vi "Dashboard Main.vi"() -> ()   [LabVIEW 2017]
uses:
  <vilib>/Utility/miscctls.llb/LVRowAndColumnTypeDef.ctl
  <vilib>/event_ctls.llb/eventvkey.ctl
  <vilib>/Rock Robotics/Network Tables/NT Read Numeric Array.vi
  <vilib>/Rock Robotics/Network Tables/NT Read Boolean.vi
  <vilib>/Rock Robotics/WPI/Dashboard/WPI_DashboardLogging Global.vi
  <vilib>/vision/NI_Vision_Development_Module.lvlib
panel:
  in  "Camera Settings Right":T1={"Frame Rate"=30, "Compression"=30, "Size"=1, "DB Camera Config"=FALSE} {"Frame Rate" scale=1.0..30.0; "Compression" scale=100.0..-1.0; "Size" items=["640x480", "320x240", "160x120"]}
  in  "Camera Name Right":string(combo)="No Camera Selection"
  out "Camera Info":cluster{"Mbps LED":bool, "Mbps":dbl, "fps":dbl} {"fps" format="%#.1g"; "Mbps" format="%#.1g"}
  in  "Camera Settings":T1={"Frame Rate"=30, "Compression"=30, "Size"=1, "DB Camera Config"=FALSE} {"Frame Rate" scale=1.0..30.0; "Compression" scale=100.0..-1.0; "Size" items=["640x480", "320x240", "160x120"]}
  in  "TCP":refnum<k5>
  in  "Rec Mode":enum32{"Stop", "Record", "Playback"}(radio)
  out "Robot IP":string
  out "Image Message":string="Timeout in Camera Communications"
  in  "Dashboard Tab":T2(tab)
  in  "Select Auto":string(combo)="Select Autonomous ..."
  out "NT Connection":bool
  out "MotorChart R":cluster{"Numeric":dbl, "Numeric":dbl}(graph)
  out "MotorChart L":cluster{"Numeric":dbl, "Numeric":dbl}(graph)
  out "MotorSliders R":cluster{"MotorSlide1":dbl, "MotorSlide2":dbl} {"MotorSlide2" scale=-1.0..1.0 scale format="%#_2e"; "MotorSlide1" scale=-1.0..1.0 scale format="%#_2e"}
  out "MotorSliders L":cluster{"MotorSlide1":dbl, "MotorSlide2":dbl} {"MotorSlide2" scale=-1.0..1.0 scale format="%#_2e"; "MotorSlide1" scale=-1.0..1.0 scale format="%#_2e"}
  out "Gyro":dbl(knob) scale=0.0..360.0
  out "JS1 Z":dbl(slide) scale=-1.0..1.0 scale format="%#_2e"
  out "JS1 Graph":cluster{"X":dbl, "Y":dbl}[](graph)
  out "JS1 Buttons":T3
  out "JS2 Z":dbl(slide) scale=-1.0..1.0 scale format="%#_2e"
  out "JS2 Graph":cluster{"X":dbl, "Y":dbl}[](graph)
  out "JS2 Buttons":T3
  out "Mode":T4(ring)=enum."Auto Disabled"
  out "Camera Image Right":T5(plugin-control)
  in  "DB/String 9":string
  in  "DB/String 8":string
  in  "DB/String 7":string
  in  "DB/String 6":string
  in  "DB/String 5":string
  in  "DB/String 4":string
  in  "DB/String 3":string
  in  "DB/String 2":string
  in  "DB/String 1":string
  in  "DB/String 0":string
  in  "DB/Slider 0":dbl(slide) scale=0.0..5.0
  in  "DB/Slider 1":dbl(slide) scale=0.0..5.0
  in  "DB/Slider 2":dbl(slide) scale=0.0..5.0
  in  "DB/Slider 3":dbl(slide) scale=0.0..5.0
  out "DB/LED 3":bool
  out "DB/LED 2":bool
  out "DB/LED 1":bool
  out "DB/LED 0":bool
  in  "DB/Button 3":bool
  in  "DB/Button 2":bool
  in  "DB/Button 1":bool
  in  "DB/Button 0":bool caption="New Name"
  out "UseLeftEncoder":bool
  out "RDrive Encoder":dbl
  out "Flip Active":bool
  in  "BackCamera Rotate":sgl min=-360 max=360 step=1 format="%#_3g"
  in  "FrontCamera Rotate":sgl min=-360 max=360 step=1 format="%#_3g"
  out "Arm Sensor":bool
  out "Belly Sensor":bool
  out "Arm Encoder":dbl
  out "Arm Switch":bool
  out "LDrive Encoder":dbl
  in  "Test Slider":dbl(slide) scale=0.0..100.0 scale format="%#_3g"
  in  "On/Off":bool caption="Solenoid"
  in  "Test Name":u16(ring) items=["Select the test to run..."]
  in  "Test Tree":string(tree)
  in  "Motor":cluster{"Value":dbl, "Enable":bool} {"Value" scale=-1.0..1.0 scale format="%#_3g"}
  out "Progress":T6 {"Test Progress" scale=0.0..100.0}
  in  "Rev/Fwd":cluster{"Forward":bool, "Reverse":bool}
  in  "Test Ring":u16(ring) items=["Monochrome", "Color"]
  out "Cmd Status":string
  in  "Execute Command":bool
  in  "Command Params":string[][](table)
  in  "Command Selection":i32(listbox)
  in  "CheckList":i32(listbox)
  out "Tree":string(tree)
  out "Camera Image":T5(plugin-control)
  out "Background":bool
  in  "Camera Name":string(combo)="No Camera Selection"
  # "HW"
  # "HW"
  # "Joysticks"
  # "Drive Motors"
  # "Front"
  # "Right"
  # "Left"
  # "Back"
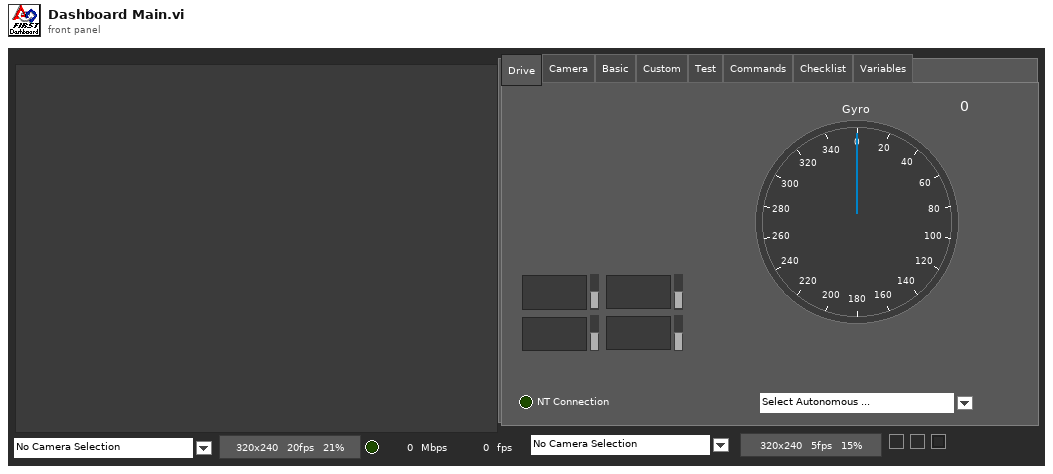
[diagram p1: front panel]
types:
  T1 = cluster{"Frame Rate":i32, "Compression":i32, "Size":u16, "DB Camera Config":bool}
  T2 = enum32{"Drive", "Camera", "Basic", "Custom", "Test", "Commands", "Checklist", "Variables"}
  T3 = cluster{bool, bool, bool, bool, bool, bool, bool, bool, bool, bool, bool, bool}
  T4 = enum8{"Tele-Op Disabled", "Tele-Op Enabled", "Auto Disabled", "Auto Enabled", "Test Disabled", "Test Enabled", "Disconnected", "No Code", "E-Stop"}
  T5 = typedef "IMAQ Image.ctl" = refnum<image>
  T6 = cluster{"Test Progress":u8, "Test Progress Text":string}
  T7 = cluster{"Save Path":path, "Interval (s)":dbl, "Keep":i32}
  T8 = typedef "Image Type" = u32
  T9 = cluster{"IDs":cluster{"RPC field ID":u16, "Unique ID":u16}, "String":string}
  T10 = cluster{string, string, "Saved DB Images Info":cluster{"Save Path":path, "Interval (s)":dbl, "Keep":i32}}
  T11 = cluster{"Camera Image":refnum<vi>, "Dashboard Tab":refnum<vi>, "Background":refnum<vi>, "Rec Mode":refnum<vi>, "Test Slider":refnum<vi>, "On/Off ":refnum<vi>, "Test Ring":refnum<vi>, "Rev/Fwd":refnum<vi>, "Test Name":refnum<vi>, "Motor":refnum<vi>, "Progress":refnum<vi>, "CheckList":refnum<vi>, "Tree":refnum<vi>, "Test Tree":refnum<vi>, "Command Params":refnum<vi>, "Command Selection":refnum<vi>, "Execute Command":refnum<vi>, "Cmd Status":refnum<vi>, "Camera Settings":refnum<vi>, "Camera Name":refnum<vi>, "Camera Info":refnum<vi>, "Camera Settings Right":refnum<vi>, "Camera Name Right":refnum<vi>, "Camera Image Right":refnum<vi>}
  T12 = cluster{"Error Strings":string, "Disable Counts":cluster{u16, u16}, "Rail Faults":cluster{u16, u16, u16}, "Robot IP":string, "DB Mode":u8, "Event Info":cluster{"Name":string, "Type":u8, "Number":u16, "Replay":u8}}
  T13 = cluster{"Storage":cluster{"Disk Free":u64, "RAM Block":u32, "RAM free":u32}, "CPU Utilization":cluster{"CPU % ISR":sgl, "CPU % Time Crit":sgl, "CPU % Timed Str":sgl, "CPU % High":sgl, "CPU % Above":sgl, "CPU % Normal":sgl, "CPU % Low":sgl}, "CAN":cluster{"% Bus Utilization":sgl, "Bus Off Cnt":u32, "TX_FIFO Full Cnt":u32, "Receive Error Cnt":u8, "Transmit Error Cnt":u8}, "HID":cluster{"HID Outputs":u32, "Rumble Low":u16, "Rumble High":u16}[]}
  T14 = cluster{"Status bits":cluster{"Test Mode":bool, "Autonomous":bool, "Enabled":bool, "Code Start":bool, "Brownout":bool, "Reserved 2":bool, "Reserved 3":bool, "E-Stop":bool}, "Code Trace":cluster{"Disabled":bool, "TeleOp":bool, "Auto":bool, "Test":bool}, "Controller Type":enum16{"unknown", "cRIO", "roboRio"}, "Code?":enum16{"unknown", "noCode", "code"}, "Battery V":dbl}
  T15 = cluster{"Control Bits":cluster{"TestMode":bool, "Autonomous":bool, "Enabled":bool, "FMS Present":bool, bool, bool, bool, "E-Stop":bool}, "Team Station ":u8, "Countdown":sgl, "Joystick Values":cluster{"Axes":dbl[], "Buttons":bool[], "POVs":i16[]}[]}
  T16 = cluster{"Axes":dbl[], "Buttons":bool[], "POVs":i16[]}[]
  T17 = cluster{"Axes":dbl[], "Buttons":bool[], "POVs":i16[]}
  T18 = cluster{"Buttons[0]":bool, "Buttons[1]":bool, "Buttons[2]":bool, "Buttons[3]":bool, "Buttons[4]":bool, "Buttons[5]":bool, "Buttons[6]":bool, "Buttons[7]":bool, "Buttons[8]":bool, "Buttons[9]":bool, "Buttons[10]":bool, "Buttons[11]":bool}
  T19 = cluster{"Camera Name Right":string, string, "Saved DB Images Info":cluster{"Save Path":path, "Interval (s)":dbl, "Keep":i32}}
  T20 = cluster{"Operation":enum16{"Update", "Clear"}, "Color Box":u32}[]
  T21 = typedef "eventvkey.ctl" = enum16{"ASCII", "Enter", "Return", "Shift", "Ctrl", "Alt", "Cmd", "Opt", "Caps", "NumLock", "Clear", "Break", "Up", "Down", "Left", "Right", "Insert", "Delete", "Home", "End", "PageUp", "PageDown", "Escape", "Help", "Pause", "ScrollLock", "F1", "F2", "F3", "F4", "F5", "F6", "F7", "F8", "F9", "F10", "F11", "F12", "F13", "F14", "F15", "F16", "F17", "F18", "F19", "F20", "F21", "F22", "F23", "F24", "Play", "VolumeUp", "VolumeDown", "Mute", "Two Byte Char"}
  T22 = cluster{"Image Size":bool, "Image Type":bool, "Pixel Value":bool, "ROI Information":bool, "Zoom Factor":bool}
  T23 = cluster{"Operation":enum16{"Update", "Clear"}, "Color Box":u32}
  T24 = typedef "LVRowAndColumnTypeDef.ctl" = cluster{"Row":i32, "Column":i32}
  T25 = cluster{"Shift":bool, "Ctrl":bool, "Alt":bool, "Cmd":bool, "Opt":bool}
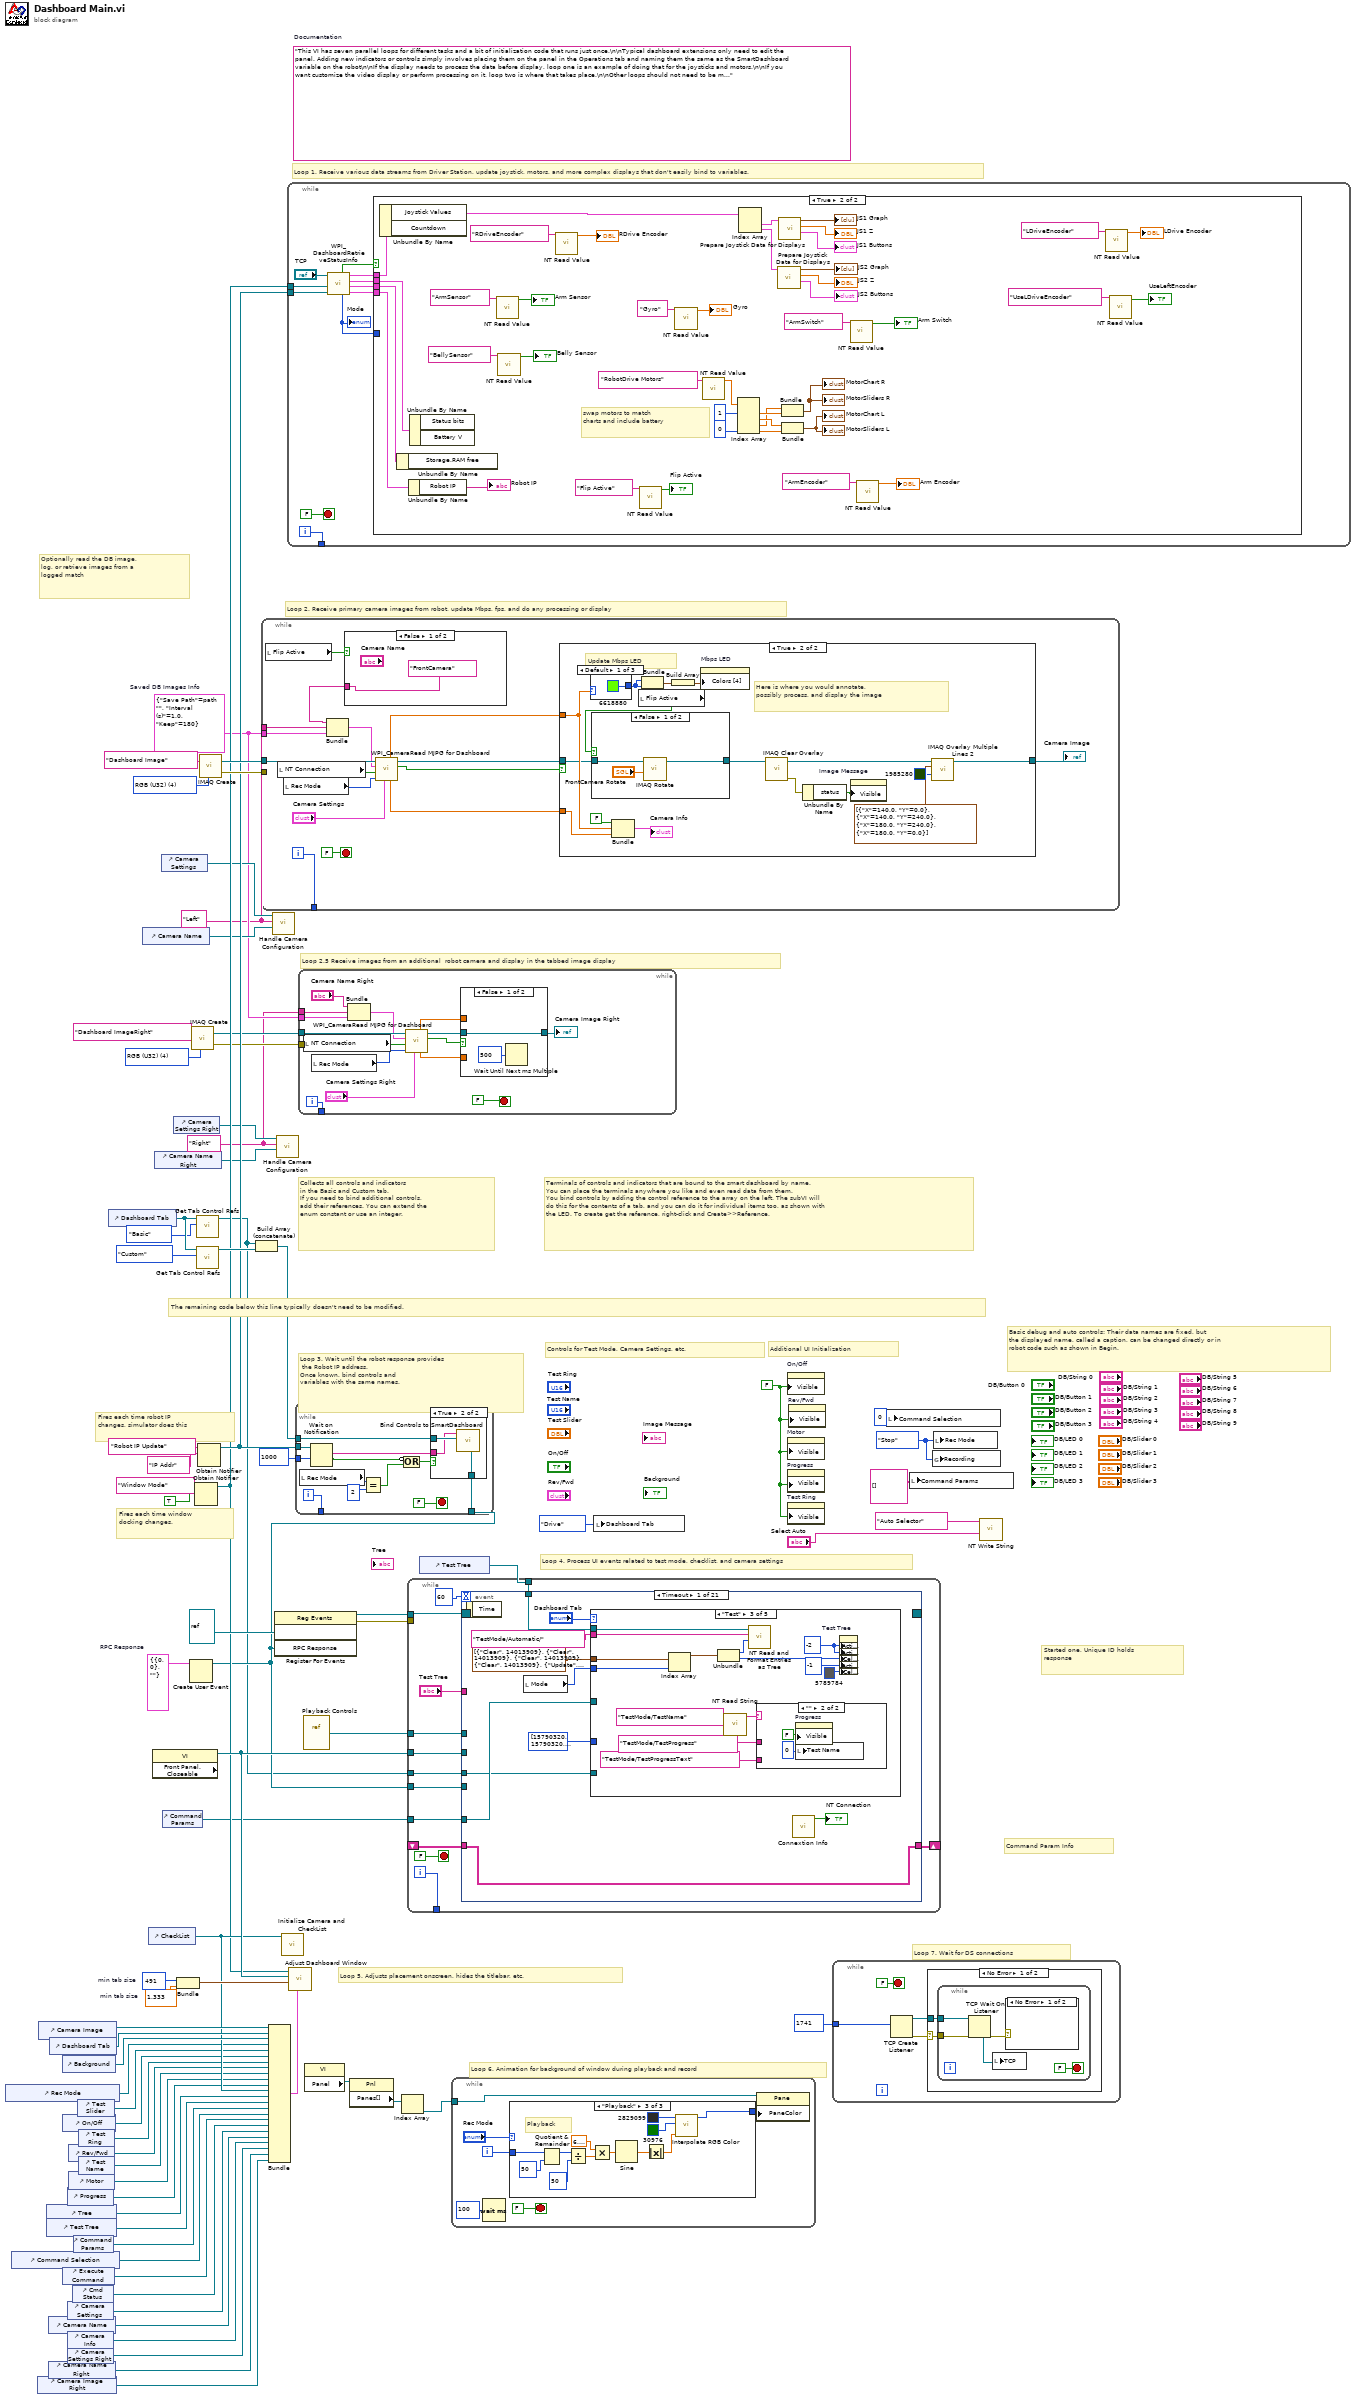
[diagram p0: block diagram]
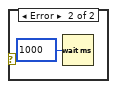
[diagram p3: hidden frame]
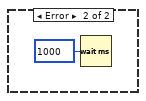
[diagram p4: hidden frame]
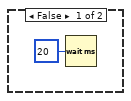
[diagram p5: hidden frame]
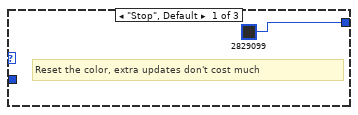
[diagram p6: hidden frame]
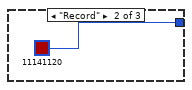
[diagram p7: hidden frame]
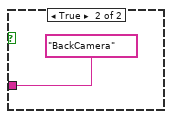
[diagram p9: hidden frame]
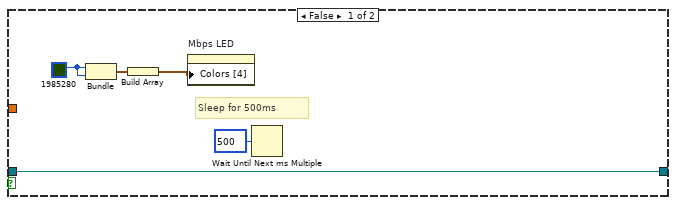
[diagram p10: hidden frame]
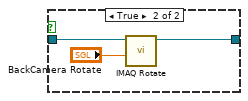
[diagram p11: hidden frame]
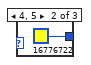
[diagram p12: hidden frame]
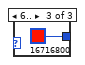
[diagram p13: hidden frame]
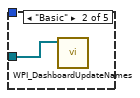
[diagram p15: hidden frame]
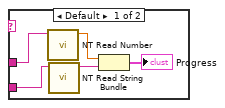
[diagram p16: hidden frame]
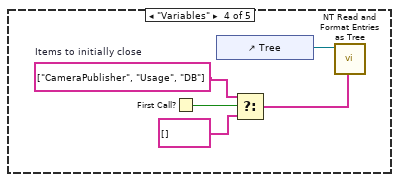
[diagram p17: hidden frame]
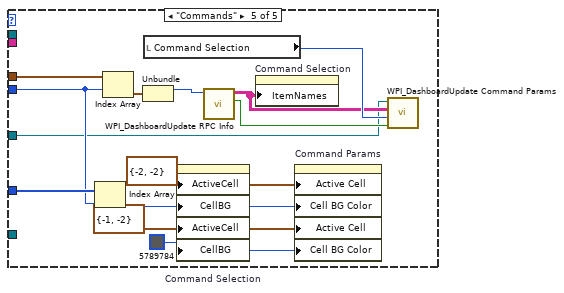
[diagram p18: hidden frame]
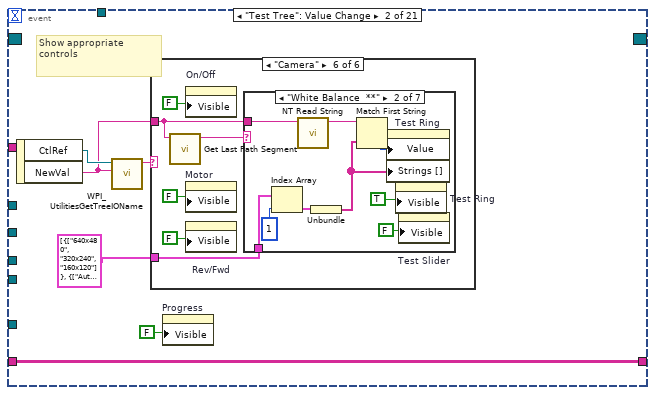
[diagram p19: hidden frame]
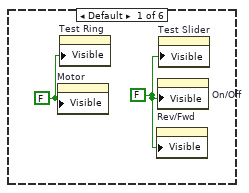
[diagram p20: hidden frame]
diagram:
  w4 = T7 {"Save Path"=path "", "Interval (s)"=1.0, "Keep"=180}  # Saved DB Images Info
  w3 = "Right"
  w2 = "Left"
  w14 = T8 4 items=["Grayscale (U8)", "Grayscale (I16)", "Grayscale (SGL)", "Complex (CSG)", "RGB (U32)", "HSL (U32)", "RGB (U64)"] ("Image Type")
  w29 = T9 {"IDs"={"RPC field ID"=0, "Unique ID"=0}, "String"=""}  # RPC Response
  w52 = 491  # min tab size
  w51 = 1.333  # min tab size
  w59 = enum32{"Stop", "Record", "Playback"}."Stop" ("Rec Mode")
  w36 = FALSE ("Visible")
  (unwired) "This VI has seven parallel loops for different tasks and a bit of initialization code that runs just once.\n\nTypical dashboard extensions only need to edit the panel. Adding new indicators or controls simply involves placing them on the panel in the Operations tab and naming them the same as the SmartDashboard variable on the robot\n\nIf the display needs to process the data before display, loop one is an example of doing that for the joysticks and motors.\n\nIf you want customize the video display or perform processing on it, loop two is where that takes place.\n\nOther loops should not need to be modified. They are pretty standard, and document the task they perform."  # Documentation
  w76 = T8 4 items=["Grayscale (U8)", "Grayscale (I16)", "Grayscale (SGL)", "Complex (CSG)", "RGB (U32)", "HSL (U32)", "RGB (U64)"] ("Image Type")
  # "Optionally read the DB image,\nlog, or retrieve images from a\nlogged match"
  # "Loop 2.5 Receive images from an additional  robot camera and display in the tabbed image display"
  # "Command Param Info"
  # "Started one, Unique ID holds\nresponse"
  # "Loop 7. Wait for DS connections"
  # "Basic debug and auto controls: Their data names are fixed, but\nthe displayed name, called a caption, can be changed directly or in\nrobot code such as shown in Begin."
  # "Controls for Test Mode, Camera Settings, etc."
  # "Additional UI Initialization"
  # "Loop 6. Animation for background of window during playback and record"
  # "Fires each time robot IP\nchanges, simulator does this"
  # "Fires each time window\ndocking changes."
  # "Collects all controls and indicators\nin the Basic and Custom tab.\nIf you need to bind additional controls,\nadd their references. You can extend the\nenum constant or use an integer."
  # "The remaining code below this line typically doesn't need to be modified."
  # "Loop 4. Process UI events related to test mode, checklist, and camera settings"
  # "Terminals of controls and indicators that are bound to the smart dashboard by name.\nYou can place the terminals anywhere you like and even read data from them.\nYou bind controls by adding the control reference to the array on the left. The subVI will\ndo this for the contents of a tab, and you can do it for individual items too, as shown with\nthe LED. To create get the reference, right-click and Create>>Reference."
  # "Loop 3. Wait until the robot response provides\n the Robot IP address.\nOnce known, bind controls and\nvariables with the same names."
  # "Loop 5. Adjusts placement onscreen, hides the titlebar, etc."
  # "Loop 1. Receive various data streams from Driver Station, update joystick, motors, and more complex displays that don't easily bind to variables."
  # "Loop 2. Receive primary camera images from robot, update Mbps, fps, and do any processing or display"
  n1 = control-ref of="Rec Mode"() -> (w42:refnum<vi>)
  n2 = control-ref of="Command Selection"() -> (w28:refnum<vi>)
  n3 = control-ref of="Camera Image Right"() -> (w7:refnum<vi>)
  n4 = control-ref of="Camera Image"() -> (w54:refnum<vi>)
  n5 = control-ref of="Tree"() -> (w46:refnum<vi>)
  n6 = control-ref of="Test Tree"() -> (w45:refnum<vi>)
  n7 = control-ref of="Camera Name"() -> (w19:refnum<vi>)
  n8 = control-ref of="Camera Name Right"() -> (w8:refnum<vi>)
  n9 = control-ref of="Dashboard Tab"() -> (w53:refnum<vi>)
  n10 = control-ref of="Execute Command"() -> (w30:refnum<vi>)
  n11 = control-ref of="Background"() -> (w49:refnum<vi>)
  n12 = control-ref of="On/Off"() -> (w40:refnum<vi>)
  n13 = control-ref of="Progress"() -> (w37:refnum<vi>)
  n14 = control-ref of="Camera Settings"() -> (w20:refnum<vi>)
  n15 = control-ref of="Camera Info"() -> (w18:refnum<vi>)
  n16 = control-ref of="Camera Settings Right"() -> (w9:refnum<vi>)
  n17 = control-ref of="Rev/Fwd"() -> (w38:refnum<vi>)
  n18 = control-ref of="Motor"() -> (w43:refnum<vi>)
  n19 = control-ref of="Cmd Status"() -> (w24:refnum<vi>)
  n20 = control-ref of="Command Params"() -> (w31:refnum<vi>)
  n21 = control-ref of="Test Slider"() -> (w41:refnum<vi>)
  n22 = control-ref of="Test Ring"() -> (w39:refnum<vi>)
  n23 = control-ref of="Test Name"() -> (w44:refnum<vi>)
  n24 = control-ref of="Dashboard Tab"() -> (w57:refnum<vi>)
  n25 = control-ref of="Camera Name"() -> (w21:refnum<vi>)
  n26 = control-ref of="CheckList"() -> (w47:refnum<vi>)
  n27 = property class="VI" props=["Front Panel.Closeable"]() -> (reference out=w58:refnum<vi>)  [unwired: 2 in, 2 out]
  n28 = control-ref of="Camera Name Right"() -> (w10:refnum<vi>)
  n29 = control-ref of="Camera Settings"() -> (w22:refnum<vi>)
  n30 = control-ref of="Command Params"() -> (w23:refnum<vi>)
  n31 = control-ref of="Camera Settings Right"() -> (w11:refnum<vi>)
  n32 = Bundle("min tab size"=w52, "min tab size"=w51) -> (w50:cluster{"min tab size":i32, "min tab size":dbl})  [unwired: 1 in]
  n33 = Create User Event(user event datatype=w29) -> (user event=w25:refnum<user-event>)  [unwired: 1 in, 1 out]
  n34 = call "IMAQ Create"("Image Name"="Dashboard ImageRight", "Image Type"=w14) -> ("New Image"=w13:T5, "error out"=w12:errorcluster)  [unwired: 2 in, 1 out]
  n35 = Obtain Notifier(name (unnamed)="Window Mode", notification data type=TRUE) -> (notifier out=w34:refnum<notifier>)  [unwired: 2 in, 2 out]
  n36 = call <vilib>:"Get Tab Control Refs.vi"("Page Index"=T2."Basic" ("Dashboard Tab"), "TabControl in"=w57) -> ("ControlsOnPage"=w17:refnum<vi>[])  [unwired: 9 in]
  n37 = call <vilib>:"Get Tab Control Refs.vi"("Page Index"=T2."Custom" ("Dashboard Tab"), "TabControl in"=w57) -> ("ControlsOnPage"=w56:refnum<vi>[])  [unwired: 9 in]
  n38 = Obtain Notifier(name (unnamed)="Robot IP Update", notification data type="IP Addr" ("name (unnamed)")) -> (notifier out=w35:refnum<notifier>)  [unwired: 2 in, 2 out]
  n39 = call "IMAQ Create"("Image Name"="Dashboard Image", "Image Type"=w76) -> ("New Image"=w74:T5, "error out"=w73:errorcluster)  [unwired: 2 in, 1 out]
  n40 = Build Array (concatenate)(w17, w56) -> (w55:refnum<vi>[])
  n41 = while {
    tunnel: w74 -> [w90]
    tunnel: w73 -> [_]
    tunnel: [w91] -> _
    tunnel: w4 -> [w81]
    tunnel: w2 -> [w80]
    i -> [w91]
    stop <- FALSE stop-if-true
    n42 = local read "Flip Active"() -> (w77:bool)
    n43 = local read "NT Connection"() -> (w82:bool)
    n44 = local read "Rec Mode"() -> (w86:enum32{"Stop", "Record", "Playback"})
    n45 = case shown="False" w77 {
      tunnel: ["FrontCamera" "BackCamera"] -> w79
      frame False {
      }
      frame True {
      }
    }
    n46 = Bundle(w79, w80, "Saved DB Images Info"=w81) -> (w78:T10)  [unwired: 1 in]
    n47 = call <vilib>:"WPI_CameraRead MJPG for Dashboard.vi"("Camera Settings"="Camera Settings", "Rec Mode"=w86, "NT Connection"=w82, "Capture Info"=w78, "Refnum in"=w90) -> ("Active"=w88:bool, "Refnum out"=w89:T5, "FPS"=w87:dbl, "Bandwidth (Mbps)"=w85:dbl)  [unwired: 3 in]
    n48 = case shown="True" w88 {
      tunnel: w89 -> [w95 w102]
      tunnel: w85 -> [_ w109]
      tunnel: w87 -> [_ w110]
      tunnel: [w95 w105] -> w83
      frame False {
        w97 = u32 1985280 ("Color Box")
        # "Sleep for 500ms"
        n49 = Bundle("Color Box"=w97, "Color Box"=w97) -> (w98:cluster{"Color Box":u32, "Color Box":u32})  [unwired: 1 out]
        n50 = Build Array(w98) -> (w96:cluster{"Color Box":u32, "Color Box":u32}[])
        n51 = property on="Mbps LED" class="Bool (strict)"("Colors [4]"=w96) -> ()  [unwired: 2 in, 2 out]
        n52 = Wait Until Next ms Multiple(millisecond multiple=u32 500) -> ()  [unwired: 1 out]
      }
      frame True {
        # "Here is where you would annotate,\npossibly process, and display the image"
        # "Update Mbps LED"
        n53 = case shown="Default" w109 {
          tunnel: [u32 6618880 ("Color Box") u32 16776722 ("Color Box") u32 16716800 ("Color Box")] -> w112
          frame Default {
          }
          frame 4, 5 {
          }
          frame 6.. {
          }
        }
        n54 = Bundle(FALSE, "Bandwidth (Mbps)"=w109, "FPS"=w110) -> (→"Camera Info":cluster{bool, "Bandwidth (Mbps)":dbl, "FPS":dbl})  [unwired: 1 in]
        n55 = local read "Flip Active"() -> (w100:bool)
        n56 = case shown="False" w100 {
          tunnel: w102 -> [w118 w121]
          tunnel: [w117 w120] -> w101
          frame False {
            n57 = call "IMAQ Rotate"("Angle (degrees)"="FrontCamera Rotate", "Image Src"=w118) -> ("Image Dst Out"=w117:T5)  [unwired: 8 in, 1 out]
          }
          frame True {
            n58 = call "IMAQ Rotate"("Angle (degrees)"="BackCamera Rotate", "Image Src"=w121) -> ("Image Dst Out"=w120:T5)  [unwired: 8 in, 1 out]
          }
        }
        n59 = Bundle("Color Box"=w112, "Color Box"=w112) -> (w113:cluster{"Color Box":u32, "Color Box":u32})  [unwired: 1 out]
        n60 = Build Array(w113) -> (w111:cluster{"Color Box":u32, "Color Box":u32}[])
        n61 = property on="Mbps LED" class="Bool (strict)"("Colors [4]"=w111) -> ()  [unwired: 2 in, 2 out]
        n62 = call "IMAQ Clear Overlay"("Image"=w101) -> ("error out"=w114:errorcluster, "Image Out"=w106:T5)  [unwired: 2 in, 7 out]
        n63 = Unbundle By Name(w114) -> ("status"=w115:bool)
        n64 = property on="Image Message" class="Str"("Visible"=w115) -> ()  [unwired: 2 in, 2 out]
        n65 = call "IMAQ Overlay Multiple Lines 2"("Image"=w106, "Line End Points"=cluster{"X":dbl, "Y":dbl}[] [{"X"=140.0, "Y"=0.0}, {"X"=140.0, "Y"=240.0}, {"X"=180.0, "Y"=240.0}, {"X"=180.0, "Y"=0.0}], "Color"=u32 1985280) -> ("Image Out"=w105:T5)  [unwired: 11 in, 1 out]
      }
    }
    "Camera Image" <- w83
  }
  n66 = Bundle("Camera Image"=w54, "Dashboard Tab"=w53, "Background"=w49, "Rec Mode"=w42, "Test Slider"=w41, "On/Off"=w40, "Test Ring"=w39, "Rev/Fwd"=w38, "Test Name"=w44, "Motor"=w43, "Progress"=w37, "CheckList"=w47, "Tree"=w46, "Test Tree"=w45, "Command Params"=w31, "Command Selection"=w28, "Execute Command"=w30, "Cmd Status"=w24, "Camera Settings"=w20, "Camera Name"=w19, "Camera Info"=w18, "Camera Settings Right"=w9, "Camera Name Right"=w8, "Camera Image Right"=w7) -> (w48:T11)  [unwired: 1 in]
  n67 = call "Handle Camera Configuration.vi"("CameraNameRef"=w21, "Display Name"=w2, "ClusterRef"=w22) -> ()  [unwired: 9 in]
  n68 = register-events(refnum<vi> refnum, w25) -> (reference out=w63:refnum<event-registration>, error out=w62:errorcluster)  [unwired: 2 in]
  n69 = call "Handle Camera Configuration.vi"("CameraNameRef"=w10, "Display Name"=w3, "ClusterRef"=w11) -> ()  [unwired: 9 in]
  n70 = call "Initialize Camera and CheckList.vi"("ListBox in"=w47) -> ()  [unwired: 11 in]
  n71 = while {
    tunnel: [w134] -> _
    tunnel: w35 -> [w128]
    tunnel: w34 -> [w125]
    i -> [w134]
    stop <- FALSE stop-if-true
    n72 = call <vilib>:"WPI_DashboardRetrieveStatusInfo.vi"("Binding Refnum"=w128, "Window Mode Notifier"=w125, "TCP Cnx"="TCP") -> ("Power and Errors"=w129:T12, "Robot Metrics"=w132:T13, "Status Info"=w133:T14, "Control Info"=w130:T15, "Robot Mode"=w127:T4, "Process?"=w131:bool)  [unwired: 3 in]
    "Mode" <- w127
    n73 = case shown="True" w131 {
      tunnel: w133 -> [_ w178]
      tunnel: w132 -> [_ w177]
      tunnel: w130 -> [_ w176]
      tunnel: w129 -> [_ w175]
      tunnel: w127 -> [_ _]
      frame False {
        n74 = Wait (ms)(milliseconds to wait=u32 20) -> ()  [unwired: 1 out]
      }
      frame True {
        # "swap motors to match\ncharts and include battery"
        n75 = Unbundle By Name(w176) -> ("Joystick Values"=w166:T16)  [unwired: 1 out]
        n76 = Unbundle By Name(w177) -> ()  [unwired: 1 out]
        n77 = Unbundle By Name(w175) -> ("Robot IP"=→"Robot IP":string)
        n78 = Unbundle By Name(w178) -> ()  [unwired: 2 out]
        n79 = call-poly <vilib>:"NT Read Value.vi"("Name"="ArmSensor") -> ("Boolean"=→"Arm Sensor":bool)  [unwired: 9 in, 1 out]
        n80 = call-poly <vilib>:"NT Read Value.vi"("Name"="BellySensor") -> ("Boolean"=→"Belly Sensor":bool)  [unwired: 9 in, 1 out]
        n81 = call-poly <vilib>:"NT Read Value.vi"("Name"="RDriveEncoder") -> ("Numeric"=→"RDrive Encoder":dbl)  [unwired: 9 in, 1 out]
        n82 = call-poly <vilib>:"NT Read Value.vi"("Name"="Flip Active") -> ("Boolean"=→"Flip Active":bool)  [unwired: 9 in, 1 out]
        n83 = call-poly <vilib>:"NT Read Value.vi"("Name"="Gyro") -> ("Numeric"=→"Gyro":dbl)  [unwired: 9 in, 1 out]
        n84 = call-poly <vilib>:"NT Read Value.vi"("Name"="RobotDrive Motors") -> ("Numeric Array"=w156:dbl[])  [unwired: 9 in, 1 out]
        n85 = Index Array(array=w156, index #1=1, index #4=0) -> (element #1=w170:dbl, element #2=w171:dbl, element #3=w169:dbl, element #4=w174:dbl)  [unwired: 2 in]
        n86 = Index Array(array=w166) -> (element #1=w165:T17, element #2=w161:T17)  [unwired: 2 in]
        n87 = call "Prepare Joystick Data for Displays.vi"("Joystick Values"=w161) -> ("Buttons"=→"JS2 Buttons":T18, "Z Axis"=→"JS2 Z":dbl, "Cartesian Data"=→"JS2 Graph":cluster{"X axis":dbl, "X axis":dbl}[])  [unwired: 8 in]
        n88 = call "Prepare Joystick Data for Displays.vi"("Joystick Values"=w165) -> ("Buttons"=→"JS1 Buttons":T18, "Z Axis"=→"JS1 Z":dbl, "Cartesian Data"=→"JS1 Graph":cluster{"X axis":dbl, "X axis":dbl}[])  [unwired: 8 in]
        n89 = Bundle("Numeric"=w169, "Numeric"=w170) -> (→"MotorChart R" →"MotorSliders R":cluster{"Numeric":dbl, "Numeric":dbl})  [unwired: 1 in]
        n90 = Bundle("Numeric"=w171, "Numeric"=w174) -> (→"MotorChart L" →"MotorSliders L":cluster{"Numeric":dbl, "Numeric":dbl})  [unwired: 1 in]
        n91 = call-poly <vilib>:"NT Read Value.vi"("Name"="ArmSwitch") -> ("Boolean"=→"Arm Switch":bool)  [unwired: 9 in, 1 out]
        n92 = call-poly <vilib>:"NT Read Value.vi"("Name"="ArmEncoder") -> ("Numeric"=→"Arm Encoder":dbl)  [unwired: 9 in, 1 out]
        n93 = call-poly <vilib>:"NT Read Value.vi"("Name"="LDriveEncoder") -> ("Numeric"=→"LDrive Encoder":dbl)  [unwired: 9 in, 1 out]
        n94 = call-poly <vilib>:"NT Read Value.vi"("Name"="UseLDriveEncoder") -> ("Boolean"=→"UseLeftEncoder":bool)  [unwired: 9 in, 1 out]
      }
    }
  }
  n95 = call "Adjust Dashboard Window.vi"("Sizing Refnums"=w48, "Size Constraints"=w50, "VI"=w58, "WIn Mode"=w34) -> ()  [unwired: 8 in]
  n96 = while {
    tunnel: w55 -> [w190]
    tunnel: w35 -> [w188]
    tunnel: [w186] -> _
    tunnel: u32 1000 ("milliseconds to wait") -> [w185]
    tunnel: w25 -> [w179]
    i -> [w186]
    stop <- FALSE stop-if-true
    n97 = local read "Rec Mode"() -> (w181:enum32{"Stop", "Record", "Playback"})
    n98 = Wait on Notification(notifier=w188, timeout in ms (-1)=w185) -> (notification=w187:string, timed out?=w183:bool)  [unwired: 2 in, 2 out]
    n99 = Equal?(x=w181, y=u16 2 ("Rec Mode")) -> (x = y?=w182:bool)
    n100 = Compound Arithmetic op=OR(invert w183, w182) -> (w184:bool)
    n101 = case shown="True" w184 {
      tunnel: w190 -> [_ w193]
      tunnel: w187 -> [_ w192]
      tunnel: w179 -> [_ w191]
      frame False {
      }
      frame True {
        n102 = call <vilib>:"Bind Controls to SmartDashboard.vi"("RPC ref"=w191, "Bound Control Refs"=w193, "Server IP Address"=w192) -> ()  [unwired: 9 in]
      }
    }
  }
  n103 = while {
    tunnel: w13 -> [w208]
    tunnel: w12 -> [_]
    tunnel: [w203] -> _
    tunnel: w4 -> [w197]
    tunnel: w3 -> [w194]
    i -> [w203]
    stop <- FALSE stop-if-true
    n104 = local read "NT Connection"() -> (w198:bool)
    n105 = local read "Rec Mode"() -> (w207:enum32{"Stop", "Record", "Playback"})
    n106 = Bundle("Camera Name Right"="Camera Name Right", w194, "Saved DB Images Info"=w197) -> (w196:T19)  [unwired: 1 in]
    n107 = call <vilib>:"WPI_CameraRead MJPG for Dashboard.vi"("Camera Settings"="Camera Settings Right", "Rec Mode"=w207, "NT Connection"=w198, "Capture Info"=w196, "Refnum in"=w208) -> ("Active"=w202:bool, "Refnum out"=w205:T5, "FPS"=w200:dbl, "Bandwidth (Mbps)"=w201:dbl)  [unwired: 3 in]
    n108 = case shown="False" w202 {
      tunnel: w205 -> [w209 w211]
      tunnel: w201 -> [_ _]
      tunnel: w200 -> [_ _]
      tunnel: [w209 w211] -> w199
      frame False {
        n109 = Wait Until Next ms Multiple(millisecond multiple=u32 500) -> ()  [unwired: 1 out]
      }
      frame True {
      }
    }
    "Camera Image Right" <- w199
  }
  n110 = vi-ref "Playback Controls.vi"() -> (w64:refnum<vi>)
  n111 = property class="VI"() -> ("Panel"=w66:refnum<vi>)  [unwired: 2 in, 2 out]
  n112 = property class="Pnl"(reference=w66) -> ("Panes[]"=w67:refnum<vi>[])  [unwired: 1 in, 2 out]
  n113 = Index Array(array=w67) -> (element=w65:refnum<vi>)  [unwired: 1 in]
  n114 = control-ref of="Test Tree"() -> (w68:refnum<vi>)
  n115 = while {
    tunnel: [w221] -> _
    tunnel: w68 -> [w220]
    tunnel: w64 -> [w219]
    tunnel: w63 -> [w218]
    tunnel: w62 -> [_]
    tunnel: w58 -> [w217]
    tunnel: w25 -> [w216]
    tunnel: w23 -> [w215]
    shift-right: [w214] -> _
    shift-left: _ -> [w213]
    tunnel: w17 -> [w212]
    i -> [w221]
    stop <- FALSE stop-if-true
    n116 = event shown="[0] Timeout" {
      selector: w218 -> [_ _ _ _ _ _ _ _ _ _ _ _ _ _ _ _ _ _ _ _ _]
      dyn-events: [_ _ _ _ _ _ _ _ _ _ _ _ _ _ _ _ w481 _ _ _ _] -> _
      timeout: u32 60 ("milliseconds to wait") -> [_ _ _ _ _ _ _ _ _ _ _ _ _ _ _ _ _ _ _ _ _]
      tunnel: w220 -> [w233 _ _ _ _ _ _ _ _ _ _ _ _ _ _ _ _ _ _ _ _]
      tunnel: "Test Tree" -> [_ _ _ _ _ _ _ _ _ _ _ w448 w456 w458 w462 w470 _ _ _ _ _]
      tunnel: w219 -> [_ _ _ _ _ _ _ _ _ _ _ _ _ _ _ _ w483 _ w501 _ _]
      tunnel: w217 -> [_ _ _ _ _ _ _ _ _ _ _ _ _ _ _ _ w479 _ _ _ _]
      tunnel: w216 -> [_ _ _ _ _ _ _ _ _ _ _ _ _ _ _ _ w477 _ _ _ _]
      tunnel: w215 -> [w228 _ _ _ _ _ w399 _ _ _ _ _ _ _ _ _ _ _ _ _ _]
      tunnel: [w227 w276 w378 w383 w392 w396 w397 w406 w416 w423 w435 w447 w454 w457 w461 w469 w476 w496 w498 w502 w515] -> w214
      tunnel: w213 -> [w227 w276 w378 w383 w392 w396 w397 _ _ w423 w435 w447 w454 w457 w461 w469 w476 w496 w498 w502 w515]
      tunnel: w212 -> [w225 _ _ _ _ _ _ _ _ _ _ _ _ _ _ _ _ _ _ _ _]
      event Timeout {
        n117 = event-data() -> ()  [unwired: 1 in, 1 out]
        n118 = local read "Mode"() -> (w230:T4)
        n119 = case shown="\"Test\"" "Dashboard Tab" {
          tunnel: w233 -> [_ _ w249 _ _]
          tunnel: "TestMode/Automatic/" ("Name Pattern") -> [_ _ w248 _ _]
          tunnel: T20 [{"Operation"=enum."Clear", "Color Box"=14013909}, {"Operation"=enum."Clear", "Color Box"=14013909}, {"Operation"=enum."Clear", "Color Box"=14013909}, {"Operation"=enum."Clear", "Color Box"=14013909}, {"Operation"=enum."Update", "Color Box"=14013909}, {"Operation"=enum."Update", "Color Box"=16777215}, {"Operation"=enum."Clear", "Color Box"=14013909}, {"Operation"=enum."Clear", "Color Box"=14013909}, {"Operation"=enum."Clear", "Color Box"=14013909}] -> [_ _ w241 _ w269]
          tunnel: w230 -> [_ _ w240 _ w268]
          tunnel: u32[] [15790320, 15790320, 15790320, 15790320, 16777215, 16777215, 15790320, 15790320, 15790320] -> [_ _ _ _ w274]
          tunnel: w228 -> [_ _ _ _ w262]
          tunnel: w225 -> [_ w235 _ _ _]
          frame "Custom", Default {
          }
          frame "Basic" {
            n120 = call <vilib>:"WPI_DashboardUpdateNames.vi"("Controls on Tab"=w235) -> ()  [unwired: 11 in]
          }
          frame "Test" {
            w247 = -2 ("Active Item:Row Number")
            n121 = Index Array(array=w241, index=w240) -> (element=w242:T23)
            n122 = Unbundle(w242) -> ("Operation"=w243:enum16{"Update", "Clear"}, "Color Box"=w244:u32)
            n123 = call <vilib>:"NT Read String.vi"("Name"="TestMode/TestName") -> ("String"=w238:string)  [unwired: 9 in, 1 out]
            n124 = call <vilib>:"NT Read and Format Entries as Tree.vi"("Operation"=w243, "Name Pattern"=w248, "Tree Refnum"=w249) -> ()  [unwired: 7 in, 2 out]
            n125 = case shown="\"\"" w238 {
              tunnel: "TestMode/TestProgress" ("Name") -> [w251 _]
              tunnel: "TestMode/TestProgressText" ("Name") -> [w250 _]
              frame Default {
                n126 = call <vilib>:"NT Read Number.vi"("Name"=w251) -> ("Numeric"=w252:dbl)  [unwired: 9 in, 1 out]
                n127 = call <vilib>:"NT Read String.vi"("Name"=w250) -> ("String"=w253:string)  [unwired: 9 in, 1 out]
                n128 = Bundle("Numeric"=w252, "String"=w253) -> (→"Progress":cluster{"Numeric":dbl, "String":string})  [unwired: 1 in]
              }
              frame "" {
                n129 = local write "Test Name"(u16 0) -> ()
                n130 = property on="Progress" class="Clust (strict)"("Visible"=FALSE) -> ()  [unwired: 2 in, 2 out]
              }
            }
            n131 = property on="Test Tree" class="Tree (strict)"("Active Item Row Number"=w247, "ActiveColNum"=w247, "CellBG"=w244, "Active Item Row Number"=-1 ("Active Item:Row Number"), "CellBG"=u32 5789784 ("Color Box")) -> ()  [unwired: 2 in, 2 out]
          }
          frame "Variables" {
            w259 = string[] ["CameraPublisher", "Usage", "DB"]  # Items to initially close
            n132 = First Call?() -> (First Call?: T/F=w260:bool)
            n133 = control-ref of="Tree"() -> (w261:refnum<vi>)
            n134 = Select(t=w259, s=w260, f=string[] []) -> (s? t:f=w257:string[])
            n135 = call <vilib>:"NT Read and Format Entries as Tree.vi"("Tags to  Close"=w257, "Tree Refnum"=w261) -> ()  [unwired: 8 in, 2 out]
          }
          frame "Commands" {
            w270 = u32 5789784 ("Color Box")
            w271 = T24 {"Row"=-1, "Column"=-2} ("Active Cell:Active Cell")
            w273 = T24 {"Row"=-2, "Column"=-2} ("Active Cell:Active Cell")
            n136 = Index Array(array=w274, index=w268) -> (element=w272:u32)
            n137 = Index Array(array=w269, index=w268) -> (element=w267:T23)
            n138 = Unbundle(w267) -> ("Operation"=w266:enum16{"Update", "Clear"})  [unwired: 1 out]
            n139 = local read "Command Selection"() -> (w265:i32)
            n140 = property on="Command Selection" class="MCListbox (strict)"("ActiveCell"=w273, "CellBG"=w272, "ActiveCell"=w271, "CellBG"=w270) -> ()  [unwired: 2 in, 2 out]
            n141 = call <vilib>:"WPI_DashboardUpdate RPC Info.vi"("Operation"=w266) -> ("update"=w264:bool, "commands"=w263:string[][])  [unwired: 9 in]
            n142 = property on="Command Selection" class="MCListbox (strict)"("ItemNames"=w263) -> ()  [unwired: 2 in, 2 out]
            n143 = property on="Command Params" class="Tbl (strict)"("Active Cell"=w273, "Cell BG Color"=w272, "Active Cell"=w271, "Cell BG Color"=w270) -> ()  [unwired: 2 in, 2 out]
            n144 = call <vilib>:"WPI_DashboardUpdate Command Params.vi"("Update"=w264, "NewVal"=w265, "Commands"=w263, "Param Tbl"=w262) -> ()  [unwired: 7 in, 1 out]
          }
        }
        n145 = call <vilib>:"Connextion Info.vi"() -> ("Connected"=→"NT Connection":bool)  [unwired: 10 in, 1 out]
      }
      event "Test Tree": Value Change {
        # "Show appropriate\ncontrols"
        n146 = event-data() -> ("CtlRef"=w279:refnum<vi>, "NewVal"=w277:string)  [unwired: 1 in]
        n147 = call <vilib>:"WPI_UtilitiesGetTreeIOName.vi"("NewVal"=w277, "TreeControl in"=w279) -> ("I/O Name"=w280:string)  [unwired: 9 in]
        n148 = case shown="\"Camera\"" w280 {
          selector: w280 -> [_ w287 _ w309 w318 _]
          tunnel: w277 -> [_ _ w306 w308 _ w325]
          tunnel: cluster{string[]}[] [{["640x480", "320x240", "160x120"]}, {["Auto", "Fixed indoor", "Fixed outdoor 1", "Fixed outdoor 2", "Fixed fluorescent 1", "Fixed fluorescent 2", "Hold current"]}, {["Auto", "Flicker-free 50 Hz", "Flicker-free 60 Hz", "Hold current"]}, {["None", "Prioritize frame rate", "Prioritize image quality"]}, {["Monochrome", "Color"]}] -> [_ _ _ _ _ w324]
          frame Default {
            w282 = FALSE ("Visible")
            w281 = FALSE ("Visible")
            n149 = property on="Motor" class="Clust (strict)"("Visible"=w281) -> ()  [unwired: 2 in, 2 out]
            n150 = property on="Test Ring" class="Ring (strict)"("Visible"=w281) -> ()  [unwired: 2 in, 2 out]
            n151 = property on="Rev/Fwd" class="Clust (strict)"("Visible"=w282) -> ()  [unwired: 2 in, 2 out]
            n152 = property on="On/Off" class="Bool (strict)"("Visible"=w282) -> ()  [unwired: 2 in, 2 out]
            n153 = property on="Test Slider" class="Slide (strict)"("Visible"=w282) -> ()  [unwired: 2 in, 2 out]
          }
          frame "Analog Out", "Motor", "PWM" {
            w288 = FALSE ("Visible")
            n154 = case shown="\"Analog Out\"" w287 {
              tunnel: [1.0 ("Value") -1.0 ("Value") 0.0 ("Value")] -> w286
              tunnel: [255.0 ("Value") 1.0 ("Value") 5.0 ("Value")] -> w285
              tunnel: [128.0 ("Value") 0.0 ("Value") 0.0 ("Value")] -> w284
              tunnel: [64.0 ("Value") 0.5 ("Value") 1.0 ("Value")] -> w283
              frame "PWM" {
              }
              frame "Motor", Default {
              }
              frame "Analog Out" {
              }
            }
            n155 = property on="Motor" class="Clust (strict)"("Visible"=TRUE) -> ()  [unwired: 2 in, 2 out]
            n156 = property on="Value" class="Slide (strict)"("Value"=w284, "Scale.Minimum"=w286, "Scale.Maximum"=w285, "Scale.Increment"=w283) -> ()  [unwired: 2 in, 2 out]
            n157 = property on="On/Off" class="Bool (strict)"("Visible"=w288) -> ()  [unwired: 2 in, 2 out]
            n158 = property on="Test Slider" class="Slide (strict)"("Visible"=w288) -> ()  [unwired: 2 in, 2 out]
            n159 = property on="Test Ring" class="Ring (strict)"("Visible"=w288) -> ()  [unwired: 2 in, 2 out]
            n160 = property on="Rev/Fwd" class="Clust (strict)"("Visible"=w288) -> ()  [unwired: 2 in, 2 out]
          }
          frame "Servo" {
            w304 = FALSE ("Visible")
            n161 = call <vilib>:"NT Read Number.vi"("Name"=w306) -> ("Numeric"=w305:dbl)  [unwired: 9 in, 1 out]
            n162 = property on="Test Slider" class="Slide (strict)"("Visible"=TRUE, "Scale.Maximum"=170.0 ("Scale.Range:Maximum")) -> ()  [unwired: 2 in, 2 out]
            n163 = local write "Test Slider"(w305) -> ()
            n164 = property on="Motor" class="Clust (strict)"("Visible"=w304) -> ()  [unwired: 2 in, 2 out]
            n165 = property on="Rev/Fwd" class="Clust (strict)"("Visible"=w304) -> ()  [unwired: 2 in, 2 out]
            n166 = property on="On/Off" class="Bool (strict)"("Visible"=w304) -> ()  [unwired: 2 in, 2 out]
            n167 = property on="Test Ring" class="Ring (strict)"("Visible"=w304) -> ()  [unwired: 2 in, 2 out]
          }
          frame "Relay", "Solenoid" {
            w307 = FALSE ("Visible")
            n168 = property on="Motor" class="Clust (strict)"("Visible"=w307) -> ()  [unwired: 2 in, 2 out]
            n169 = property on="Test Slider" class="Slide (strict)"("Visible"=w307) -> ()  [unwired: 2 in, 2 out]
            n170 = Search and Replace String(input string=w308, search string="/Value  **", replace string="/Direction") -> (result string=w314:string)  [unwired: 5 in, 3 out]
            n171 = property on="Test Ring" class="Ring (strict)"("Visible"=w307) -> ()  [unwired: 2 in, 2 out]
            n172 = call <vilib>:"NT Read String.vi"("Name"=w314) -> ("String"=w312:string)  [unwired: 9 in, 1 out]
            n173 = Equal?(x="Both directions", y=w312) -> (x = y?=w310:bool)
            n174 = Not(x=w310) -> (.not. x?=w311:bool)
            n175 = property on="Rev/Fwd" class="Clust (strict)"("Visible"=w310) -> ()  [unwired: 2 in, 2 out]
            n176 = property on="On/Off" class="Bool (strict)"("Visible"=w311, "Caption.Text"=w309) -> ()  [unwired: 2 in, 2 out]
          }
          frame "Compressor", "Digital Out" {
            w317 = FALSE ("Visible")
            # "Get direction and finish"
            n177 = property on="Motor" class="Clust (strict)"("Visible"=w317) -> ()  [unwired: 2 in, 2 out]
            n178 = property on="Test Slider" class="Slide (strict)"("Visible"=w317) -> ()  [unwired: 2 in, 2 out]
            n179 = property on="Test Ring" class="Ring (strict)"("Visible"=w317) -> ()  [unwired: 2 in, 2 out]
            n180 = property on="On/Off" class="Bool (strict)"("Visible"=TRUE, "Caption.Text"=w318) -> ()  [unwired: 2 in, 2 out]
            n181 = property on="Rev/Fwd" class="Clust (strict)"("Visible"=FALSE) -> ()  [unwired: 2 in, 2 out]
          }
          frame "Camera" {
            n182 = call <vilib>:"Get Last Path Segment.vi"("String in"=w325) -> ("String out"=w326:string)  [unwired: 10 in]
            n183 = property on="On/Off" class="Bool (strict)"("Visible"=FALSE) -> ()  [unwired: 2 in, 2 out]
            n184 = property on="Motor" class="Clust (strict)"("Visible"=FALSE) -> ()  [unwired: 2 in, 2 out]
            n185 = property on="Rev/Fwd" class="Clust (strict)"("Visible"=FALSE) -> ()  [unwired: 2 in, 2 out]
            n186 = case shown="\"White Balance  **\"" w326 {
              tunnel: w325 -> [w332 w341 w350 w359 w368 _ w374]
              tunnel: w324 -> [w330 w338 w347 w356 w365 _ _]
              frame "Size  **" {
                n187 = Index Array(array=w330) -> (element=w329:cluster{string[]})  [unwired: 1 in]
                n188 = call <vilib>:"NT Read String.vi"("Name"=w332) -> ("String"=w331:string)  [unwired: 9 in, 1 out]
                n189 = Unbundle(w329) -> (w327:string[])
                n190 = Match First String(2:w327, 3:w331) -> (0:w328:i32)  [unwired: 1 out]
                n191 = property on="Test Ring" class="Ring (strict)"("Value"=w328, "Strings []"=w327) -> ()  [unwired: 2 in, 2 out]
                n192 = property on="Test Ring" class="Ring (strict)"("Visible"=TRUE) -> ()  [unwired: 2 in, 2 out]
                n193 = property on="Test Slider" class="Slide (strict)"("Visible"=FALSE) -> ()  [unwired: 2 in, 2 out]
              }
              frame "White Balance  **" {
                n194 = Index Array(array=w338, index=1) -> (element=w339:cluster{string[]})
                n195 = call <vilib>:"NT Read String.vi"("Name"=w341) -> ("String"=w340:string)  [unwired: 9 in, 1 out]
                n196 = Unbundle(w339) -> (w336:string[])
                n197 = Match First String(2:w336, 3:w340) -> (0:w335:i32)  [unwired: 1 out]
                n198 = property on="Test Ring" class="Ring (strict)"("Value"=w335, "Strings []"=w336) -> ()  [unwired: 2 in, 2 out]
                n199 = property on="Test Ring" class="Ring (strict)"("Visible"=TRUE) -> ()  [unwired: 2 in, 2 out]
                n200 = property on="Test Slider" class="Slide (strict)"("Visible"=FALSE) -> ()  [unwired: 2 in, 2 out]
              }
              frame "Exposure  **" {
                n201 = Index Array(array=w347, index=2) -> (element=w348:cluster{string[]})
                n202 = call <vilib>:"NT Read String.vi"("Name"=w350) -> ("String"=w349:string)  [unwired: 9 in, 1 out]
                n203 = Unbundle(w348) -> (w344:string[])
                n204 = Match First String(2:w344, 3:w349) -> (0:w345:i32)  [unwired: 1 out]
                n205 = property on="Test Ring" class="Ring (strict)"("Value"=w345, "Strings []"=w344) -> ()  [unwired: 2 in, 2 out]
                n206 = property on="Test Ring" class="Ring (strict)"("Visible"=TRUE) -> ()  [unwired: 2 in, 2 out]
                n207 = property on="Test Slider" class="Slide (strict)"("Visible"=FALSE) -> ()  [unwired: 2 in, 2 out]
              }
              frame "Exposure Priority  **" {
                n208 = Index Array(array=w356, index=3) -> (element=w357:cluster{string[]})
                n209 = call <vilib>:"NT Read String.vi"("Name"=w359) -> ("String"=w358:string)  [unwired: 9 in, 1 out]
                n210 = Unbundle(w357) -> (w353:string[])
                n211 = Match First String(2:w353, 3:w358) -> (0:w354:i32)  [unwired: 1 out]
                n212 = property on="Test Ring" class="Ring (strict)"("Value"=w354, "Strings []"=w353) -> ()  [unwired: 2 in, 2 out]
                n213 = property on="Test Ring" class="Ring (strict)"("Visible"=TRUE) -> ()  [unwired: 2 in, 2 out]
                n214 = property on="Test Slider" class="Slide (strict)"("Visible"=FALSE) -> ()  [unwired: 2 in, 2 out]
              }
              frame "Color Enable  **" {
                n215 = Index Array(array=w365, index=4) -> (element=w366:cluster{string[]})
                n216 = call <vilib>:"NT Read String.vi"("Name"=w368) -> ("String"=w367:string)  [unwired: 9 in, 1 out]
                n217 = Unbundle(w366) -> (w362:string[])
                n218 = Match First String(2:w362, 3:w367) -> (0:w363:i32)  [unwired: 1 out]
                n219 = property on="Test Ring" class="Ring (strict)"("Value"=w363, "Strings []"=w362) -> ()  [unwired: 2 in, 2 out]
                n220 = property on="Test Ring" class="Ring (strict)"("Visible"=TRUE) -> ()  [unwired: 2 in, 2 out]
                n221 = property on="Test Slider" class="Slide (strict)"("Visible"=FALSE) -> ()  [unwired: 2 in, 2 out]
              }
              frame Default {
                n222 = property on="Test Ring" class="Ring (strict)"("Visible"=FALSE) -> ()  [unwired: 2 in, 2 out]
                n223 = property on="Test Slider" class="Slide (strict)"("Visible"=FALSE) -> ()  [unwired: 2 in, 2 out]
              }
              frame "Brightness  **", "Color Level  **", "Compression  **", "FPS  **", "Sharpness  **" {
                n224 = call <vilib>:"NT Read Number.vi"("Name"=w374) -> ("Numeric"=w373:dbl)  [unwired: 9 in, 1 out]
                n225 = local write "Test Slider"(w373) -> ()
                n226 = property on="Test Slider" class="Slide (strict)"("Visible"=TRUE, "Scale.Maximum"=100.0 ("Scale.Range:Maximum")) -> ()  [unwired: 2 in, 2 out]
                n227 = property on="Test Ring" class="Ring (strict)"("Visible"=FALSE) -> ()  [unwired: 2 in, 2 out]
              }
            }
          }
        }
        n228 = property on="Progress" class="Clust (strict)"("Visible"=FALSE) -> ()  [unwired: 2 in, 2 out]
      }
      event "Test Name": Mouse Enter {
        # "Populate the ring with the list of tests"
        n229 = event-data() -> ()  [unwired: 1 in, 1 out]
        n230 = call <vilib>:"NT Read String Array.vi"("Name"="TestMode/TestList") -> ("String Array"=w382:string[])  [unwired: 9 in, 1 out]
        n231 = Build Array (concatenate)("Select the test to run...", w382) -> (w381:string[])
        n232 = property on="Test Name" class="Ring (strict)"("Strings []"=w381) -> ()  [unwired: 2 in, 2 out]
      }
      event "Test Name": Value Change {
        w384 = FALSE ("Visible")
        # "Tell the robot the test name to run"
        n233 = event-data() -> ("NewVal"=w388:u16)  [unwired: 1 in]
        n234 = property on="Test Name" class="Ring (strict)"() -> ("Strings []"=w389:string[])  [unwired: 2 in, 2 out]
        n235 = local write "Progress"(T6 {"Test Progress"=0, "Test Progress Text"=""} ("Progress")) -> ()
        n236 = Index Array(array=w389, index=w388) -> (element=w387:string)
        n237 = call <vilib>:"NT Write String.vi"("String"=w387, "Name"="TestMode/TestName") -> ()  [unwired: 9 in, 1 out]
        n238 = property on="Progress" class="Clust (strict)"("Visible"=TRUE) -> ()  [unwired: 2 in, 2 out]
        n239 = property on="Motor" class="Clust (strict)"("Visible"=w384) -> ()  [unwired: 2 in, 2 out]
        n240 = property on="Test Slider" class="Slide (strict)"("Visible"=w384) -> ()  [unwired: 2 in, 2 out]
        n241 = property on="On/Off" class="Bool (strict)"("Visible"=w384) -> ()  [unwired: 2 in, 2 out]
        n242 = property on="Rev/Fwd" class="Clust (strict)"("Visible"=w384) -> ()  [unwired: 2 in, 2 out]
        n243 = property on="Test Ring" class="Ring (strict)"("Visible"=w384) -> ()  [unwired: 2 in, 2 out]
      }
      event "Select Auto": Mouse Enter {
        # "Populate the combo box with the list of autonomous options"
        n244 = event-data() -> ()  [unwired: 1 in, 1 out]
        n245 = call <vilib>:"NT Read String Array.vi"("Name"="Auto List2") -> ("String Array"=w391:string[])  [unwired: 9 in, 1 out]
        n246 = property on="Select Auto" class="CmbBox"("Strings[]"=w391) -> ()  [unwired: 2 in, 2 out]
      }
      event "Select Auto": Value Change {
        # "User modified the Auto Selection. Write to NT variable so robot knows."
        n247 = event-data() -> ("NewVal"=w394:string)  [unwired: 1 in]
        n248 = call <vilib>:"NT Write String.vi"("String"=w394, "Name"="Auto Selector") -> ()  [unwired: 9 in, 1 out]
      }
      event "Command Selection": Value Change {
        # "Get the params and show in table"
        n249 = event-data() -> ("NewVal"=w400:i32)  [unwired: 1 in]
        n250 = property on="Command Selection" class="MCListbox (strict)"() -> ("ItemNames"=w398:string[][])  [unwired: 2 in, 2 out]
        n251 = call <vilib>:"WPI_DashboardUpdate Command Params.vi"("NewVal"=w400, "Commands"=w398, "Param Tbl"=w399) -> ()  [unwired: 8 in, 1 out]
      }
      event "Execute Command": Value Change {
        # "Started one, Unique ID holds\nresponse"
        n252 = event-data() -> ()  [unwired: 1 in, 1 out]
        n253 = property on="Command Selection" class="MCListbox (strict)"() -> ("ItemNames"=w411:string[][])  [unwired: 2 in, 2 out]
        n254 = Index Array(array=w411, index (row)="Command Selection", index (col)=0) -> (element=w409:string)
        n255 = call <vilib>:"Invoke Commands.vi"("Command Params"="Command Params", "Function Name"=w409) -> ("Params"=w405:u8, "Started"=w404:bool)  [unwired: 7 in, 1 out]
        n256 = Array Subset(array="Command Params", length (row)=w405) -> (w406:string[][])  [unwired: 3 in]
        n257 = Select(t="Executing" ("Cmd Status"), s=w404, f="" ("Cmd Status")) -> (s? t:f=→"Cmd Status":string)
      }
      event "Command Selection": Double Click {
        n258 = event-data() -> ("Row"=w419:i32)  [unwired: 1 in]
        n259 = local read "Command Params"() -> (w418:string[][])
        n260 = property on="Command Selection" class="MCListbox (strict)"() -> ("ItemNames"=w422:string[][])  [unwired: 2 in, 2 out]
        n261 = Index Array(array=w422, index (row)=w419, index (col)=0) -> (element=w420:string)
        n262 = call <vilib>:"Invoke Commands.vi"("Command Params"=w418, "Function Name"=w420) -> ("Params"=w417:u8, "Started"=w412:bool)  [unwired: 7 in, 1 out]
        n263 = Array Subset(array=w418, length (row)=w417) -> (w416:string[][])  [unwired: 3 in]
        n264 = Select(t="Executing" ("Cmd Status"), s=w412, f="" ("Cmd Status")) -> (s? t:f=w413:string)
        n265 = local write "Cmd Status"(w413) -> ()
      }
      event "CheckList": Double Click {
        # "Shift clears all"
        # "Update symbols on the listbox"
        n266 = event-data() -> ("PlatMods.Shift"=w424:bool, "Row"=w426:i32)  [unwired: 1 in]
        n267 = case shown="True" w424 {
          tunnel: w426 -> [w430 _]
          tunnel: 1 -> [w429 _]
          frame False {
            n268 = property on="CheckList" class="LstBox (strict)"() -> ("Item Symbols"=w428:i32[])  [unwired: 2 in, 2 out]
            n269 = Replace Array Subset(array=w428, new element=w429, index=w430) -> (w427:i32[])
            n270 = property on="CheckList" class="LstBox (strict)"("Item Symbols"=w427) -> ()  [unwired: 2 in, 2 out]
          }
          frame True {
            w431 = 0 ("Top Row")
            n271 = property on="CheckList" class="LstBox (strict)"() -> ("Number of Rows"=w433:u32)  [unwired: 2 in, 2 out]
            n272 = Initialize Array(0, w433) -> (w432:i32[])
            n273 = property on="CheckList" class="LstBox (strict)"("Top Row"=w431, "Value"=w431, "Item Symbols"=w432) -> ()  [unwired: 2 in, 2 out]
          }
        }
      }
      event "CheckList": Key Down {
        # "Update symbols on the listbox\nLeft and right keys check and uncheck"
        n274 = event-data() -> ("VKey"=w437:T21)  [unwired: 1 in]
        n275 = case shown="\"Left\", \"Right\"" w437 {
          selector: w437 -> [w442 _]
          tunnel: eventvkey."Left" ("VKey") -> [w440 _]
          frame "Left", "Right" {
            n276 = Equal?(x=w440, y=w442) -> (x = y?=w441:bool)
            n277 = Select(t=0, s=w441, f=1) -> (s? t:f=w443:i32)
            n278 = property on="CheckList" class="LstBox (strict)"() -> ("Item Symbols"=w446:i32[])  [unwired: 2 in, 2 out]
            n279 = Replace Array Subset(array=w446, new element=w443, index="CheckList") -> (w445:i32[])
            n280 = property on="CheckList" class="LstBox (strict)"("Item Symbols"=w445) -> ()  [unwired: 2 in, 2 out]
          }
          frame Default {
          }
        }
      }
      event "Motor.Enable": Value Change {
        # "When the test mode otor enable helper is set, update that\ntree row item's value"
        n281 = event-data() -> ("NewVal"=w452:bool)  [unwired: 1 in]
        n282 = Unbundle("Motor") -> ("Value"=w451:dbl)  [unwired: 1 out]
        n283 = Select(t=w451, s=w452, f=0.0) -> (s? t:f=w449:dbl)
        n284 = call <vilib>:"NT Write Number.vi"("Numeric"=w449, "Name"=w448) -> ()  [unwired: 9 in, 1 out]
      }
      event "Test Slider": Value Change {
        # "When the test mode slider helper is set, update that\ntree row item's value"
        n285 = event-data() -> ("NewVal"=w455:dbl)  [unwired: 1 in]
        n286 = call <vilib>:"NT Write Number.vi"("Numeric"=w455, "Name"=w456) -> ()  [unwired: 9 in, 1 out]
      }
      event "On/Off": Value Change {
        # "When the test mode on/off helper value is set, update that\ntree row item's value"
        n287 = event-data() -> ("NewVal"=w460:bool)  [unwired: 1 in]
        n288 = Boolean To (0,1)(Boolean=w460) -> (0, 1=w459:i16)
        n289 = call <vilib>:"NT Write Number.vi"("Numeric"=w459, "Name"=w458) -> ()  [unwired: 9 in, 1 out]
      }
      event "Rev/Fwd": Value Change {
        # "When the test mode helper value for relays is set, update that\ntree row item's value"
        n290 = event-data() -> ("NewVal.Forward"=w468:bool, "NewVal.Reverse"=w467:bool)  [unwired: 1 in]
        n291 = Boolean To (0,1)(Boolean=w468) -> (0, 1=w464:i16)
        n292 = Boolean To (0,1)(Boolean=w467) -> (0, 1=w466:i16)
        n293 = Negate(x=w466) -> (-x=w465:i16)
        n294 = Add(x=w464, y=w465) -> (x+y=w463:i16)
        n295 = call <vilib>:"NT Write Number.vi"("Numeric"=w463, "Name"=w462) -> ()  [unwired: 9 in, 1 out]
      }
      event "Test Ring": Value Change {
        # "When a test mode helper value is selected from the ring,\nset the tree item's variable to the string value"
        n296 = event-data() -> ("NewVal"=w472:u16)  [unwired: 1 in]
        n297 = property on="Test Ring" class="Ring (strict)"() -> ("Strings []"=w473:string[])  [unwired: 2 in, 2 out]
        n298 = Index Array(array=w473, index=w472) -> (element=w471:string)
        n299 = call <vilib>:"NT Write String.vi"("String"=w471, "Name"=w470) -> ()  [unwired: 9 in, 1 out]
      }
      event "Rec Mode": Value Change {
        # "Update globals for recording mode and path to read log from.\nClear when logging and let NetworkTables set path for vision to\nuse."
        n300 = event-data() -> ("NewVal"=w484:enum32{"Stop", "Record", "Playback"})  [unwired: 1 in]
        n301 = global write "WPI_DashboardLogging Global.vi" "Logging Filename"(path "") -> ()
        n302 = global write "WPI_DashboardLogging Global.vi" "Recording"(w484) -> ()
        n303 = case shown="\"Playback\"" w484 {
          tunnel: w483 -> [_ w486 w495]
          tunnel: [_ _ w494] -> w481
          tunnel: [_ _ w493] -> _
          tunnel: w479 -> [_ _ w491]
          tunnel: cluster{i32, i32} {-250, 170} -> [_ _ w490]
          tunnel: [_ _ T22 {"Image Size"=TRUE, "Image Type"=TRUE, "Pixel Value"=TRUE, "ROI Information"=TRUE, "Zoom Factor"=FALSE} ("Image Information Shown:All Elements")] -> w474
          tunnel: [_ _ TRUE ("Zoom Factor")] -> w475
          tunnel: w477 -> [_ _ w487]
          frame Default {
          }
          frame "Stop", "Record" {
            # "Place Window too"
            n304 = invoke class="VI" method="FP.Close"(reference=w486) -> (reference out=w485:refnum<vi>)  [unwired: 2 in, 2 out]
            n305 = invoke class="VI" method="Abort VI"(reference=w485) -> ()  [unwired: 2 in, 3 out]
          }
          frame "Playback" {
            n306 = call "Open Playback Panel.vi"("Offset"=w490, "DB VI Ref"=w491, "Playback in"=w495) -> ("Playback out"=w492:refnum<vi>)  [unwired: 8 in]
            n307 = register-events(w492, w487) -> (reference out=w494:refnum<event-registration>, error out=w493:errorcluster)  [unwired: 2 in]
          }
        }
        n308 = property on="Camera Image Right" class="ImageControl"("Image Information Shown"=w474, "Image Information Visible"=w475) -> ()  [unwired: 2 in, 2 out]
        n309 = property on="Camera Image" class="ImageControl"("Image Information Shown"=w474, "Image Information Visible"=w475) -> ()  [unwired: 2 in, 2 out]
        n310 = call <vilib>:"WPI_DashboardNT Log FieldName Cache.vi"("Operation"=enum16{"Lookup/Add", "Index", "Clear"}."Clear") -> ()  [unwired: 8 in, 3 out]
      }
      event Panel Close {
        w497 = enum32{"Stop", "Record", "Playback"}."Stop" ("Rec Mode")
        # "Playback window has been closed, abort"
        n311 = event-data() -> ()  [unwired: 1 in, 4 out]
        n312 = local write "Rec Mode"(w497) -> ()
        n313 = global write "WPI_DashboardLogging Global.vi" "Recording"(w497) -> ()
      }
      event Panel Close {
        # "Abort playback window and ourself"
        n314 = event-data() -> ()  [unwired: 1 in, 4 out]
        n315 = invoke class="VI" method="FP.Close"(reference=w501) -> (reference out=w500:refnum<vi>)  [unwired: 2 in, 2 out]
        n316 = invoke class="VI" method="Abort VI"(reference=w500) -> (error out=w499:errorcluster)  [unwired: 2 in, 2 out]
        n317 = invoke class="VI" method="Abort VI"(error in=w499) -> ()  [unwired: 2 in, 3 out]
      }
      event User Event {
        n318 = event-data() -> ("IDs"=w508:cluster{"RPC field ID":u16, "Unique ID":u16}, "String"=w507:string)  [unwired: 1 in]
        n319 = Bundle("IDs"=w508, "String"=w507) -> (w506:T9)  [unwired: 1 in]
        n320 = call <vilib>:"Retrieve RPC Response.vi"("RPC Response"=w506) -> ("Output"=w504:string[][])  [unwired: 10 in]
        n321 = Build Array (concatenate)(w502, w504) -> (w503:string[][])
        n322 = local write "Command Params"(w503) -> ()
        n323 = local write "Cmd Status"("" ("Cmd Status")) -> ()
      }
      event "Tree": Double Click {
        n324 = event-data() -> ("PlatMods"=w514:T25, "Tag"=w511:string)  [unwired: 1 in]
        n325 = Unbundle(w514) -> ("Shift"=w513:bool)  [unwired: 4 out]
        n326 = String Subset(string=w511, length (rest)=1 ("length (rest)")) -> (substring=w510:string)  [unwired: 1 in]
        n327 = Not(x=w513) -> (.not. x?=w512:bool)
        n328 = case shown="\"/\"" w510 {
          tunnel: w511 -> [_ w517]
          tunnel: w512 -> [_ w516]
          frame Default {
          }
          frame "/" {
            n329 = call <vilib>:"NT Update Persistence.vi"("Persistence"=w516, "Name"=w517) -> ()  [unwired: 9 in, 1 out]
          }
        }
      }
    }
  }
  n330 = while {
    tunnel: w65 -> [w519]
    i -> [w522]
    stop <- FALSE stop-if-true
    n331 = Wait (ms)(milliseconds to wait=u32 100) -> ()  [unwired: 1 out]
    n332 = case shown="\"Playback\"" "Rec Mode" {
      tunnel: w522 -> [_ _ w537]
      tunnel: [u32 2829099 ("Base Color") u32 11141120 ("Target Color") w526] -> w518
      frame "Stop", Default {
        # "Reset the color, extra updates don't cost much"
      }
      frame "Record" {
      }
      frame "Playback" {
        # "Playback"
        n333 = Quotient & Remainder(x=w537, y=u32 50 ("milliseconds to wait")) -> (x-y*floor(x/y)=w533:u32)  [unwired: 1 out]
        n334 = Divide(x=w533, y=u32 50 ("milliseconds to wait")) -> (x/y=w530:dbl)
        n335 = Multiply(x=6.283185307179586, y=w530) -> (x*y=w535:dbl)
        n336 = Sine(x=w535) -> (sin(x)=w534:dbl)
        n337 = Absolute Value(x=w534) -> (abs(x)=w527:dbl)
        n338 = call "Interpolate RGB Color.vi"("Proportion"=w527, "Target Color"=u32 30976, "Base Color"=u32 2829099) -> ("Result Color"=w526:u32)  [unwired: 8 in]
      }
    }
    n339 = property class="Pane"(reference=w519, "PaneColor"=w518) -> ()  [unwired: 1 in, 2 out]
  }
  n340 = local write "Dashboard Tab"(T2."Drive" ("Dashboard Tab")) -> ()
  n341 = property on="On/Off" class="Bool (strict)"("Visible"=w36) -> ()  [unwired: 2 in, 2 out]
  n342 = property on="Motor" class="Clust (strict)"("Visible"=w36) -> ()  [unwired: 2 in, 2 out]
  n343 = property on="Progress" class="Clust (strict)"("Visible"=w36) -> ()  [unwired: 2 in, 2 out]
  n344 = property on="Test Ring" class="Ring (strict)"("Visible"=w36) -> ()  [unwired: 2 in, 2 out]
  n345 = property on="Rev/Fwd" class="Clust (strict)"("Visible"=w36) -> ()  [unwired: 2 in, 2 out]
  n346 = while {
    tunnel: u16 1741 ("timeout ms (25000)") -> [w539]
    stop <- FALSE stop-if-true
    n347 = TCP Create Listener(10:w539) -> (0:w538:errorcluster, 3:w540:refnum<k5>)  [unwired: 4 in, 1 out]
    n348 = case shown="No Error" w538 {
      selector: w538 -> [w542 _]
      tunnel: w540 -> [w543 _]
      frame No Error {
        n349 = while {
          tunnel: w543 -> [w546]
          tunnel: w542 -> [w545]
          stop <- FALSE stop-if-true
          n350 = TCP Wait On Listener(8:w545, 11:w546) -> (0:w547:errorcluster, 4:w548:refnum<k5>)  [unwired: 2 in, 3 out]
          n351 = local write "TCP"(w548) -> ()
          n352 = case shown="No Error" w547 {
            frame No Error {
            }
            frame Error {
              n353 = Wait (ms)(milliseconds to wait=u32 1000) -> ()  [unwired: 1 out]
            }
          }
        }
      }
      frame Error {
        n354 = Wait (ms)(milliseconds to wait=u32 1000) -> ()  [unwired: 1 out]
      }
    }
  }
  n355 = local write "Command Selection"(u16 0 ("milliseconds to wait")) -> ()
  n356 = local write "Command Params"(string[][] [] ("Command Params")) -> ()
  n357 = global write "WPI_DashboardLogging Global.vi" "Recording"(w59) -> ()
  n358 = local write "Rec Mode"(w59) -> ()
  n359 = call <vilib>:"NT Write String.vi"("String"="Select Auto", "Name"="Auto Selector") -> ()  [unwired: 9 in, 1 out]
